vi "KickTo.vi"(8 "error in (no error)":errorcluster, 9 "Ball":refnum<class "Ball.lvclass">, 10 "Robot":refnum<class "Robot.lvclass">, 11 "KickToSkill in":refnum<class "KickToSkill.lvclass">) -> (0 "error out":errorcluster, 2 "Robot out":refnum<class "Robot.lvclass">, 3 "KickToSkill out":refnum<class "KickToSkill.lvclass">)   [LabVIEW 2023, in "KickToSkill.lvclass"]
uses:
  KickToSkill.lvclass
  Robot_class/Robot.lvclass
  Ball_class/Ball.lvclass
  Game_class/Navigation/driveMode.ctl
  Robot_class/Robot.lvclass/Robot.ctl
  Robot_class/Write kick_x.vi
  Robot_class/Write kick_z.vi
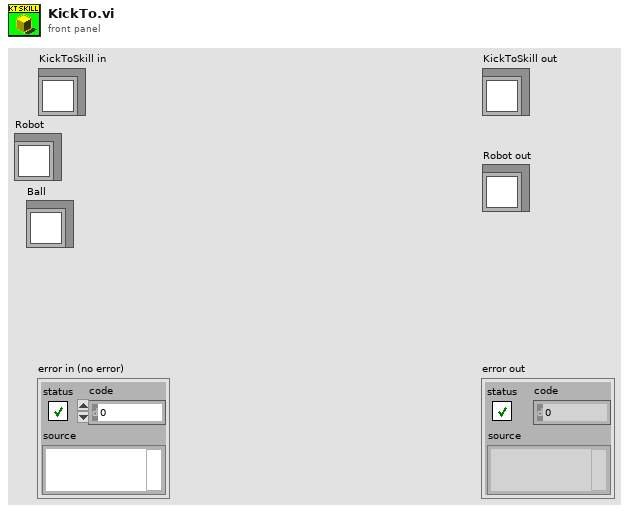
[diagram p1: front panel]
types:
  T1 = typedef "driveMode.ctl" = enum16{"Fast", "SafeDrive"}
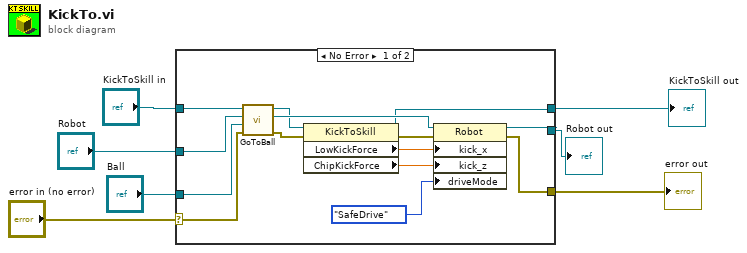
[diagram p0: block diagram]
diagram:
  n1 = case shown="No Error" "error in (no error)" {
    selector: "error in (no error)" -> [w18 w24]
    tunnel: [w11 w24] -> w6
    tunnel: [w9 w23] -> w4
    tunnel: "KickToSkill in" -> [w21 w23]
    tunnel: "Robot" -> [w20 w22]
    tunnel: "Ball" -> [w19 _]
    tunnel: [w10 w22] -> w1
    frame No Error {
      n2 = call-dynamic "GoToBall.vi"("error in (no error)"=w18, "Ball"=w19, "Robot"=w20, "GoToSkill in"=w21) -> ("error out"=w13:errorcluster, "Robot out"=w17:refnum<class "Robot.lvclass">, "GoToSkill out"=w16:refnum<class "KickToSkill.lvclass">)  [unwired: 5 in]
      n3 = property class="KickToSkill"(reference=w16, error in=w13) -> (reference out=w9:refnum<class "KickToSkill.lvclass">, error out=w12:errorcluster, "LowKickForce"=w15:dbl, "ChipKickForce"=w14:dbl)
      n4 = property class="Robot"(reference=w17, error in=w12, "kick_x"=w15, "kick_z"=w14, "driveMode"=driveMode."SafeDrive") -> (reference out=w10:refnum<class "Robot.lvclass">, error out=w11:errorcluster)
    }
    frame Error {
    }
  }
  "error out" <- w6
  "KickToSkill out" <- w4
  "Robot out" <- w1
